vi "GetPositionCategory.vi"(8 "error in (no error)":errorcluster, 11 "ClickableText in":refnum<class "ClickableText.lvclass">) -> (0 "error out":errorcluster, 2 "position":T1, 3 "ClickableText out":refnum<class "ClickableText.lvclass">)   [LabVIEW 2009, in "NavScreen.lvlib" / "ClickableText.lvclass"]
uses:
  ClickableText.lvclass
  PositionCategory.ctl
  ClickableText.lvclass/ClickableText.ctl
  NavScreen.lvlib
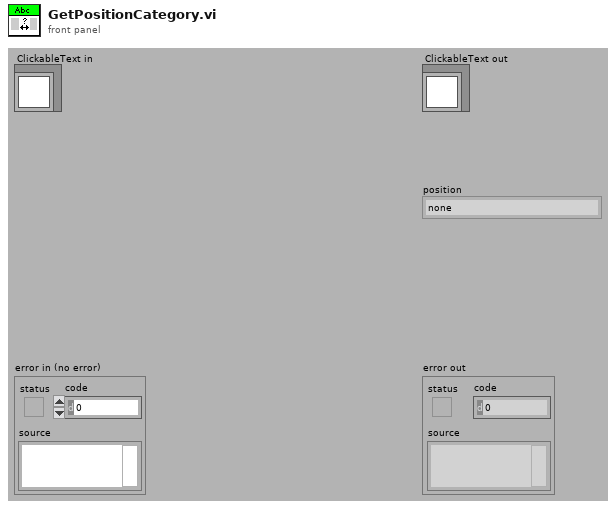
[diagram p1: front panel]
types:
  T1 = typedef "NavScreen.lvlib/PositionCategory.ctl" = enum16{"none", "column 1", "column 2", "ring"}
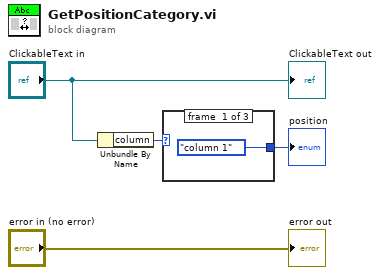
[diagram p0: block diagram]
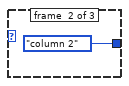
[diagram p2: hidden frame]
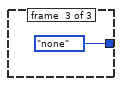
[diagram p3: hidden frame]
diagram:
  n1 = Unbundle By Name("ClickableText in") -> ("column"=w2:u8)
  n2 = case shown="Default" w2 {
    tunnel: [PositionCategory."column 1" ("position") PositionCategory."column 2" ("position") PositionCategory."none" ("position")] -> w1
    frame #0 {
    }
    frame #1 {
    }
    frame #2 {
    }
  }
  "position" <- w1
  "error out" <- "error in (no error)"
  "ClickableText out" <- "ClickableText in"
